vi "CRYSet Default Calibrate Device After Delete.vi"(8 "Deleted Calibrated Device":string, 9 "Current Signal Type":string, 10 "Input/Output":bool, 11 "Calibration In":T1 {"Calibration 2D"."Sens Curve"."Z data" items=["dB", "Lin"]; "Calibration 2D"."Sens Curve"."X data" items=["dB", "Lin"]; "Calibration 2D"."Sens Curve"."Y data" items=["dB", "Lin"]; "Calibration 2D"."Sens Curve"."Z dB ref" format="%.1f"; "Calibration 2D"."Sens Curve"."Z axis" items=["Log", "Lin"]; "Calibration 2D"."Sens Curve"."X dB ref" format="%.1f"; "Calibration 2D"."Sens Curve"."X axis" items=["Log", "Lin"]; "Calibration 2D"."Sens Curve"."Y axis" items=["Log", "Lin"]; "Calibration 2D"."Sens Curve"."Y dB ref" format="%.1f"; "Calibration 2D"."Sens Curve"."Curve"."z" format="%.2f"; "Calibration 2D"."Sens Curve"."Curve"."y" format="%.2f"; "Calibration 2D"."Sens Curve"."Curve"."x" format="%.2f"; "Calibration 2D"."EQ Curve"."Z data" items=["dB", "Lin"]; "Calibration 2D"."EQ Curve"."X data" items=["dB", "Lin"]; "Calibration 2D"."EQ Curve"."Y data" items=["dB", "Lin"]; "Calibration 2D"."EQ Curve"."Z dB ref" format="%.1f"; "Calibration 2D"."EQ Curve"."Z axis" items=["Log", "Lin"]; "Calibration 2D"."EQ Curve"."X dB ref" format="%.1f"; "Calibration 2D"."EQ Curve"."X axis" items=["Log", "Lin"]; "Calibration 2D"."EQ Curve"."Y axis" items=["Log", "Lin"]; "Calibration 2D"."EQ Curve"."Y dB ref" format="%.1f"; "Calibration 2D"."EQ Curve"."Curve"."z" format="%.2f"; "Calibration 2D"."EQ Curve"."Curve"."y" format="%.2f"; "Calibration 2D"."EQ Curve"."Curve"."x" format="%.2f"; "Calibration 2D"."Corr Curve"."Z data" items=["dB", "Lin"]; "Calibration 2D"."Corr Curve"."X data" items=["dB", "Lin"]; "Calibration 2D"."Corr Curve"."Y data" items=["dB", "Lin"]; "Calibration 2D"."Corr Curve"."Z dB ref" format="%.1f"; "Calibration 2D"."Corr Curve"."Z axis" items=["Log", "Lin"]; "Calibration 2D"."Corr Curve"."X dB ref" format="%.1f"; "Calibration 2D"."Corr Curve"."X axis" items=["Log", "Lin"]; "Calibration 2D"."Corr Curve"."Y axis" items=["Log", "Lin"]; "Calibration 2D"."Corr Curve"."Y dB ref" format="%.1f"; "Calibration 2D"."Corr Curve"."Curve"."z" format="%.2f"; "Calibration 2D"."Corr Curve"."Curve"."y" format="%.2f"; "Calibration 2D"."Corr Curve"."Curve"."x" format="%.2f"; "Calibration 2D"."Calibration"."EQ Step size" items=["R10", "R20", "R40", "R80", "User"]; "Calibration 2D"."Calibration"."Corr Step size" items=["R10", "R20", "R40", "R80", "User"]}) -> (2 "unity cal Name":string, 3 "Calibration Out":T1 {"Calibration 2D"."Sens Curve"."Z data" items=["dB", "Lin"]; "Calibration 2D"."Sens Curve"."X data" items=["dB", "Lin"]; "Calibration 2D"."Sens Curve"."Y data" items=["dB", "Lin"]; "Calibration 2D"."Sens Curve"."Z dB ref" format="%.1f"; "Calibration 2D"."Sens Curve"."Z axis" items=["Log", "Lin"]; "Calibration 2D"."Sens Curve"."X dB ref" format="%.1f"; "Calibration 2D"."Sens Curve"."X axis" items=["Log", "Lin"]; "Calibration 2D"."Sens Curve"."Y axis" items=["Log", "Lin"]; "Calibration 2D"."Sens Curve"."Y dB ref" format="%.1f"; "Calibration 2D"."Sens Curve"."Curve"."z" format="%.2f"; "Calibration 2D"."Sens Curve"."Curve"."y" format="%.2f"; "Calibration 2D"."Sens Curve"."Curve"."x" format="%.2f"; "Calibration 2D"."EQ Curve"."Z data" items=["dB", "Lin"]; "Calibration 2D"."EQ Curve"."X data" items=["dB", "Lin"]; "Calibration 2D"."EQ Curve"."Y data" items=["dB", "Lin"]; "Calibration 2D"."EQ Curve"."Z dB ref" format="%.1f"; "Calibration 2D"."EQ Curve"."Z axis" items=["Log", "Lin"]; "Calibration 2D"."EQ Curve"."X dB ref" format="%.1f"; "Calibration 2D"."EQ Curve"."X axis" items=["Log", "Lin"]; "Calibration 2D"."EQ Curve"."Y axis" items=["Log", "Lin"]; "Calibration 2D"."EQ Curve"."Y dB ref" format="%.1f"; "Calibration 2D"."EQ Curve"."Curve"."z" format="%.2f"; "Calibration 2D"."EQ Curve"."Curve"."y" format="%.2f"; "Calibration 2D"."EQ Curve"."Curve"."x" format="%.2f"; "Calibration 2D"."Corr Curve"."Z data" items=["dB", "Lin"]; "Calibration 2D"."Corr Curve"."X data" items=["dB", "Lin"]; "Calibration 2D"."Corr Curve"."Y data" items=["dB", "Lin"]; "Calibration 2D"."Corr Curve"."Z dB ref" format="%.1f"; "Calibration 2D"."Corr Curve"."Z axis" items=["Log", "Lin"]; "Calibration 2D"."Corr Curve"."X dB ref" format="%.1f"; "Calibration 2D"."Corr Curve"."X axis" items=["Log", "Lin"]; "Calibration 2D"."Corr Curve"."Y axis" items=["Log", "Lin"]; "Calibration 2D"."Corr Curve"."Y dB ref" format="%.1f"; "Calibration 2D"."Corr Curve"."Curve"."z" format="%.2f"; "Calibration 2D"."Corr Curve"."Curve"."y" format="%.2f"; "Calibration 2D"."Corr Curve"."Curve"."x" format="%.2f"; "Calibration 2D"."Calibration"."EQ Step size" items=["R10", "R20", "R40", "R80", "User"]; "Calibration 2D"."Calibration"."Corr Step size" items=["R10", "R20", "R40", "R80", "User"]})   [LabVIEW 2013]
uses:
  Typedef Control/CRYCalibration All Cluster.ctl
  Typedef Control/CRYCalibration 2DCluster.ctl
  Typedef Control/CRYCalibration Cluster.ctl
  Typedef Control/CRYData Cluster.ctl
  CRYMainGlobal.vi
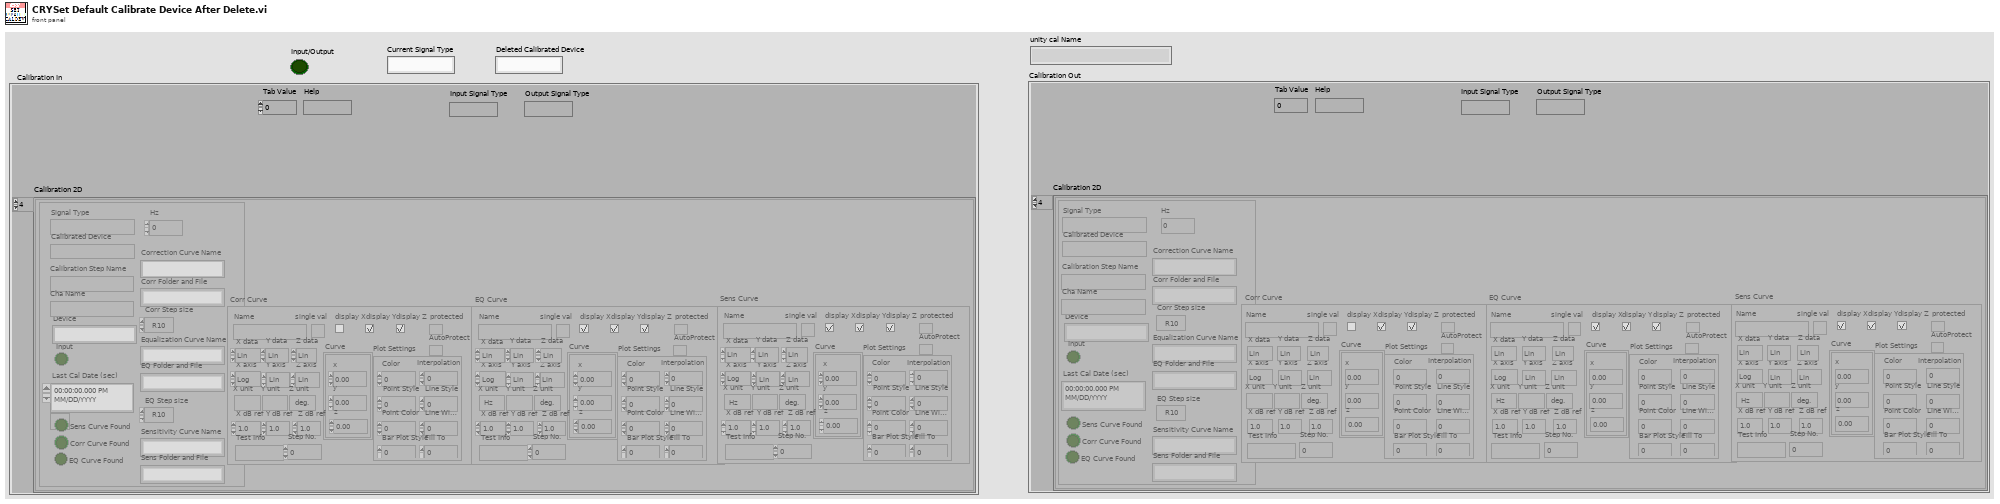
[diagram p1: front panel]
types:
  T1 = typedef "CRYCalibration All Cluster.ctl" = cluster{"Calibration 2D":T2[], "Help":string, "Tab Value":i32, "Input Signal Type":string, "Output Signal Type":string}
  T2 = typedef "CRYCalibration 2DCluster.ctl" = cluster{"Calibration":T3, "Corr Curve":T4, "EQ Curve":T4, "Sens Curve":T4}
  T3 = typedef "CRYCalibration Cluster.ctl" = cluster{"Calibration Step Name":string, "Device":string, "Correction Curve Name":string, "Equalization Curve Name":string, "Sensitivity Curve Name":string, "Corr Folder and File":string, "EQ Folder and File":string, "Sens Folder and File":string, "Corr Step size":u16, "EQ Step size":u16, "Input":bool, "Last Cal Date (sec)":timestamp, "Cha Name":string, "Corr Curve Found":bool, "EQ Curve Found":bool, "Sens Curve Found":bool, "Signal Type":string, "Calibrated Device":string, "Hz":u32}
  T4 = typedef "CRYData Cluster.ctl" = cluster{"Name":string, "Curve":cluster{"x":dbl, "y":dbl, "z":dbl}[], "X data":u16, "Y data":u16, "Z data":u16, "X axis":u16, "Y axis":u16, "Z axis":u16, "X unit":string, "Y unit":string, "Z unit":string, "X dB ref":dbl, "Y dB ref":dbl, "Z dB ref":dbl, "single val":bool, "protected":bool, "display X":bool, "display Y":bool, "display Z":bool, "Test Info":string, "Step No.":i32, "Plot Settings":cluster{"Color":u32, "Interpolation":u8, "Point Style":u8, "Line Style":u8, "Point Color":u32, "Line Width":u8, "Bar Plot Style":u8, "Fill To":i16}, "AutoProtect":bool}
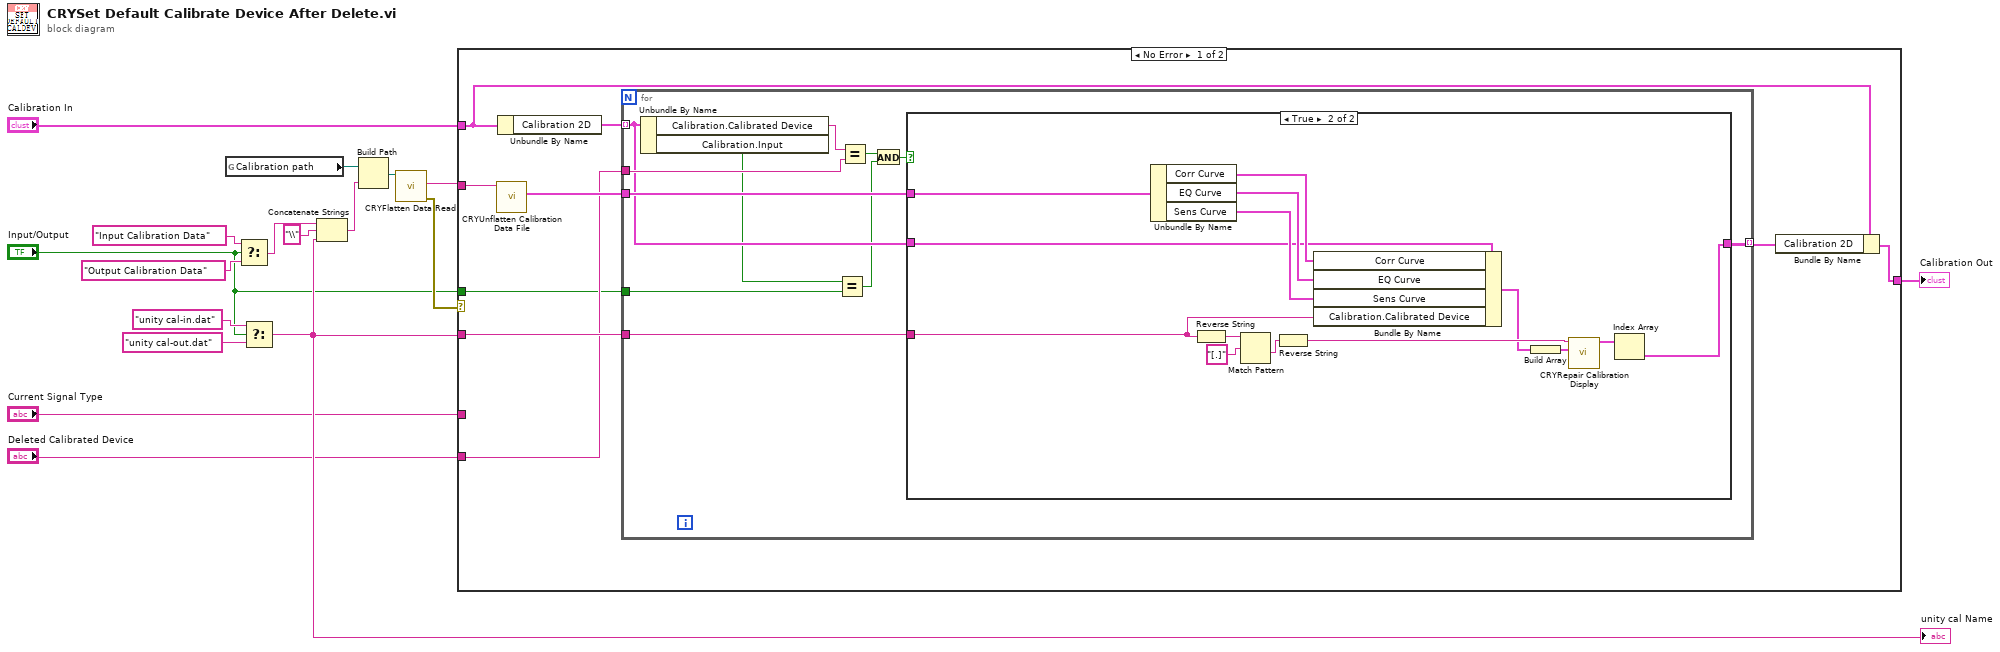
[diagram p0: block diagram]
diagram:
  n1 = global read "CRYMainGlobal.vi" "Calibration path"() -> (w16:path)
  n2 = Select(t="Input Calibration Data" ("name or relative path"), s="Input/Output", f="Output Calibration Data" ("name or relative path")) -> (s? t:f=w6:string)
  n3 = Select(t="unity cal-in.dat" ("y"), s="Input/Output", f="unity cal-out.dat" ("y")) -> (s? t:f=w7:string)
  "unity cal Name" <- w7
  n4 = Concatenate Strings(w6, "\\" ("string"), w7) -> (w13:string)
  n5 = Build Path(base path=w16, name or relative path=w13) -> (appended path=w15:path)
  n6 = call "CRYFlatten Data Read.vi"("Path In"=w15) -> ("error out"=w12:errorcluster, "Flatten Data Out"=w17:string)  [unwired: 6 in, 1 out]
  n7 = case shown="No Error" w12 {
    tunnel: w17 -> [w24 _]
    tunnel: w7 -> [w26 _]
    tunnel: "Calibration In" -> [w21 w53]
    tunnel: [w19 w53] -> w4
    tunnel: "Current Signal Type" -> [_ _]
    tunnel: "Deleted Calibrated Device" -> [w22 _]
    tunnel: "Input/Output" -> [w18 _]
    frame No Error {
      n8 = call "CRYUnflatten Calibration Data File.vi"("Flattened Calibration"=w24) -> ("Calibration 2D Data File Out"=w23:T2)  [unwired: 8 in, 2 out]
      n9 = Unbundle By Name(w21) -> ("Calibration 2D"=w25:T2[])
      n10 = for {
        tunnel: w26 -> [w37]
        tunnel: w25 -> [w33] mode=indexing
        tunnel: w23 -> [w36]
        tunnel: w22 -> [w34]
        tunnel: [w32] -> w20 mode=indexing
        tunnel: w18 -> [w31]
        n11 = Unbundle By Name(w33) -> ("Calibration.Calibrated Device"=w35:string, "Calibration.Input"=w30:bool)
        n12 = Equal?(x=w30, y=w31) -> (x = y?=w29:bool)
        n13 = Equal?(x=w35, y=w34) -> (x = y?=w28:bool)
        n14 = And(x=w28, y=w29) -> (x .and. y?=w27:bool)
        n15 = case shown="True" w27 {
          tunnel: w37 -> [_ w47]
          tunnel: w36 -> [_ w41]
          tunnel: w33 -> [w38 w40]
          tunnel: [w38 w39] -> w32
          frame False {
          }
          frame True {
            n16 = Unbundle By Name(w41) -> ("Corr Curve"=w50:T4, "EQ Curve"=w51:T4, "Sens Curve"=w52:T4)
            n17 = Reverse String(1:w47) -> (0:w46:string)
            n18 = Match Pattern(string=w46, regular expression="[.]") -> (after substring=w49:string)  [unwired: 4 out]
            n19 = Reverse String(1:w49) -> (0:w45:string)
            n20 = Bundle By Name(cluster=w40, "Corr Curve"=w50, "EQ Curve"=w51, "Sens Curve"=w52, "Calibration.Calibrated Device"=w47) -> (w44:T2)
            n21 = Build Array(w44) -> (w43:T2[])
            n22 = call "CRYRepair Calibration Display.vi"("Calibration In"=w43, "Calibration Step Name"=w45) -> ("Calibration Out"=w42:T2[])  [unwired: 1 in, 8 out]
            n23 = Index Array(array=w42) -> (element=w39:T2)  [unwired: 1 in]
          }
        }
      }
      n24 = Bundle By Name(cluster=w21, "Calibration 2D"=w20) -> (w19:T1)
    }
    frame Error {
    }
  }
  "Calibration Out" <- w4
